vi "WebServiceFGV.vi"(7 "CMD":T5, 8 "error in (no error)":errorcluster, 9 "ClientTimeout(s)(30)":dbl=30.0 format="%#_13g", 10 "ClientName":string, 11 "SRListIn":T3=[{"SR#"=0.0, "Group"="", "Owner"="", "Problem Summary"="", "Last Updated"=timestamp(0 s since 1904-01-01), "Customer First Name"="", "Customer Last Name"="", "Company"="", "Created On"=timestamp(0 s since 1904-01-01), "SR Type"="", "Status"="", "Service Level"="", "Channel"="", "Days Open"=0.0}] {"SR#" format="%#_10g"}) -> (0 "error out":errorcluster, 2 "ClientList":T1, 3 "SRListOut":T3 {"SR#" format="%#_10g"})   [LabVIEW 2017, in "Server.lvlib" / "WebServiceCommunication.lvlib"]
uses:
  WebServiceCommunication.lvlib
  WebServiceFGVcommands.ctl
  TypeDefs/SR List.ctl
  TypeDefs/SR Data.ctl
  TypeDefs/ClientList.ctl
  TypeDefs/ClientData.ctl
  WebServiceData.ctl
  Server.lvlib
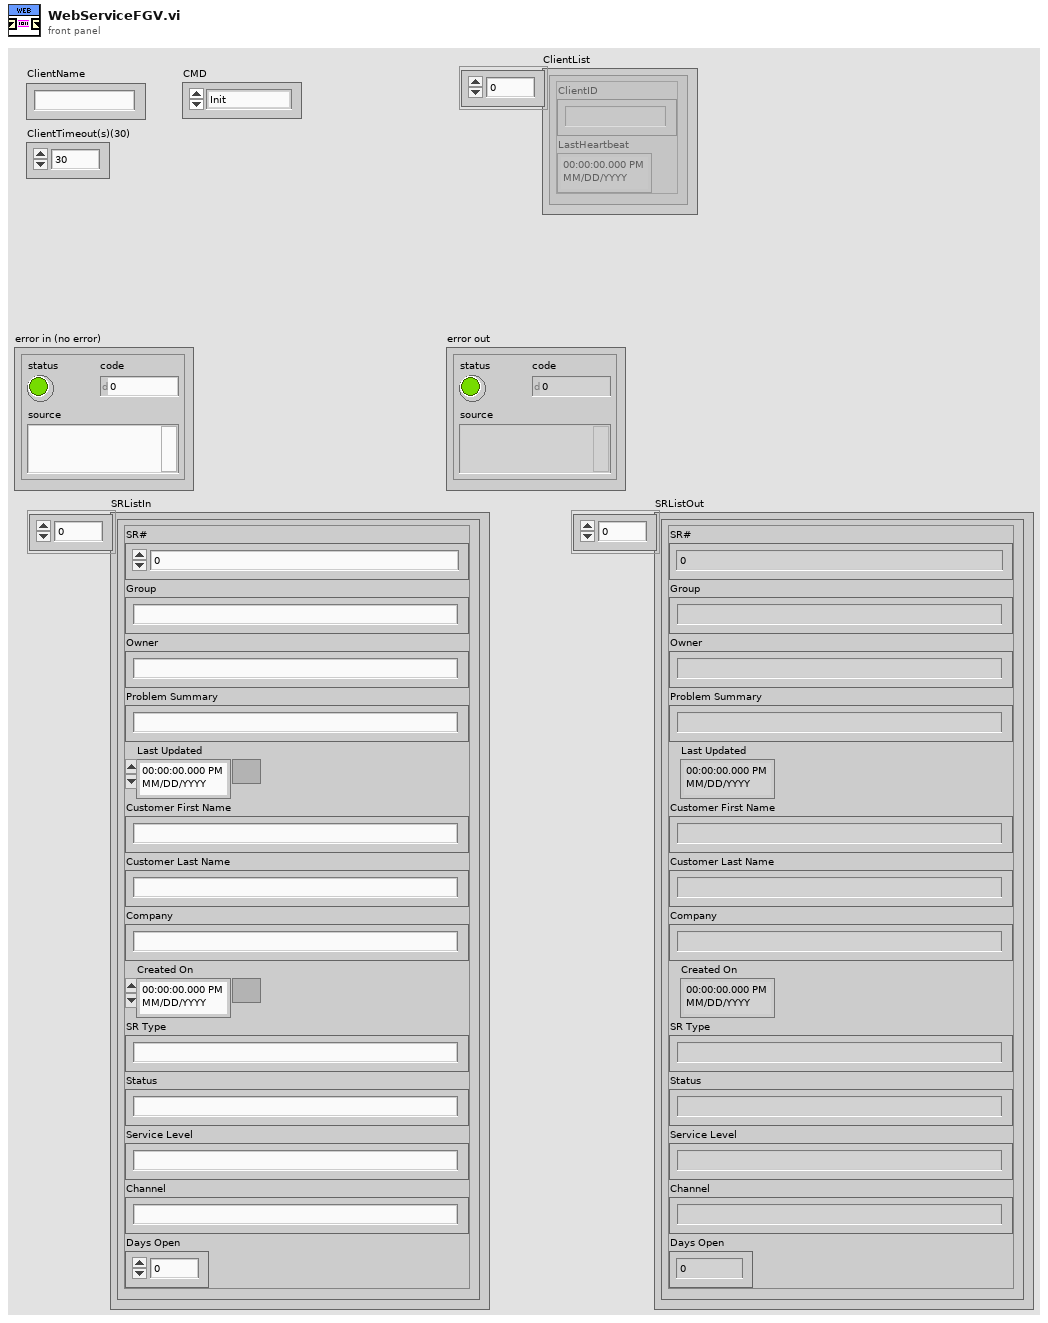
[diagram p1: front panel]
types:
  T1 = typedef "Server.lvlib/ClientList.ctl" = T2[]
  T2 = typedef "Server.lvlib/ClientData.ctl" = cluster{"ClientID":string, "LastHeartbeat":timestamp}
  T3 = typedef "Server.lvlib/SR List.ctl" = T4[]
  T4 = typedef "Server.lvlib/SR Data.ctl" = cluster{"SR#":dbl, "Group":string, "Owner":string, "Problem Summary":string, "Last Updated":timestamp, "Customer First Name":string, "Customer Last Name":string, "Company":string, "Created On":timestamp, "SR Type":string, "Status":string, "Service Level":string, "Channel":string, "Days Open":dbl}
  T5 = typedef "Server.lvlib/WebServiceCommunication.lvlib/WebServiceFGVcommands.ctl" = enum16{"Init", "Reset", "Heartbeat", "GetSRs", "SetSRs", "CheckClients", "GetClients"}
  T6 = typedef "Server.lvlib/WebServiceCommunication.lvlib/WebServiceData.ctl" = cluster{"SRList":T3, "ClientList":T1}
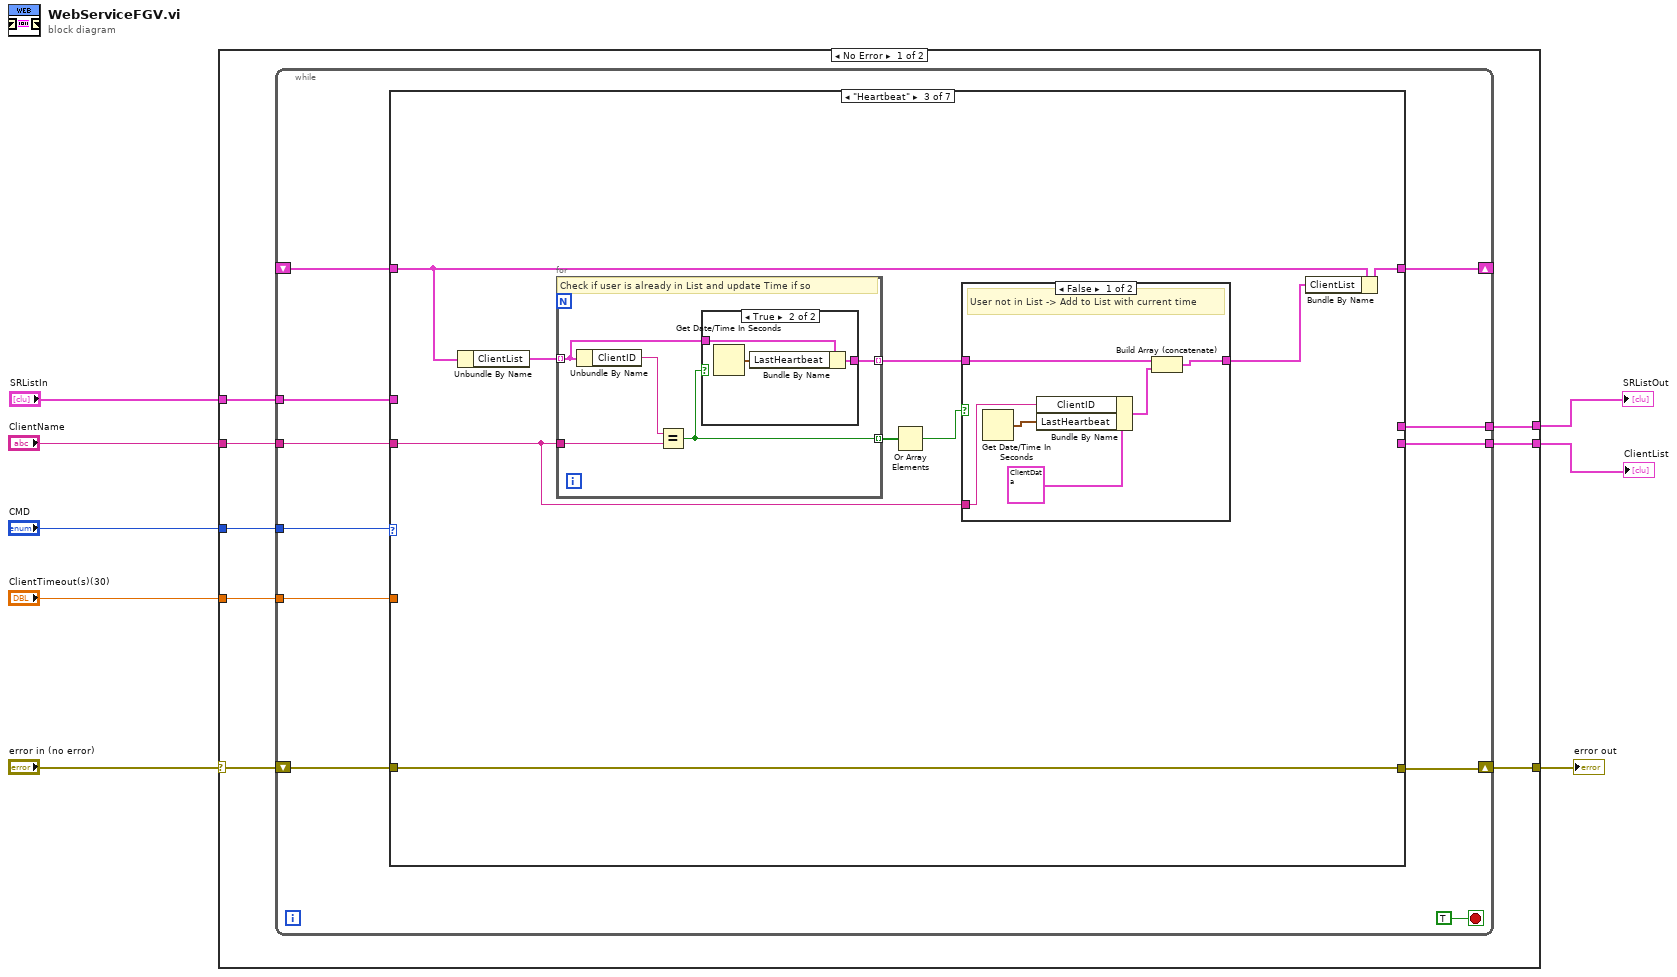
[diagram p0: block diagram]
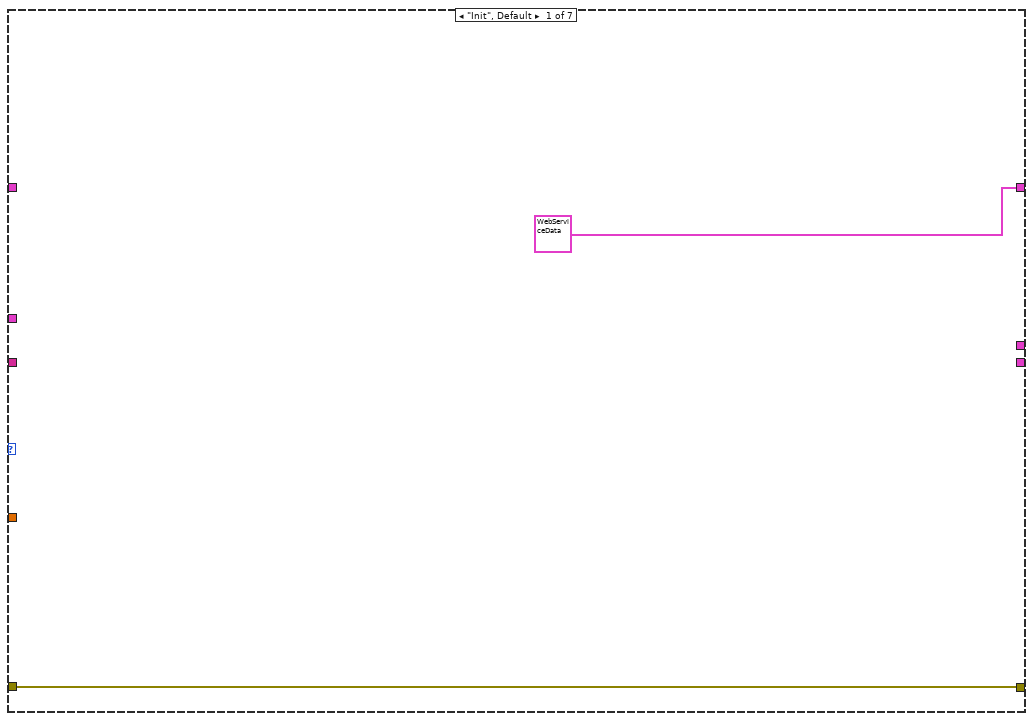
[diagram p2: hidden frame]
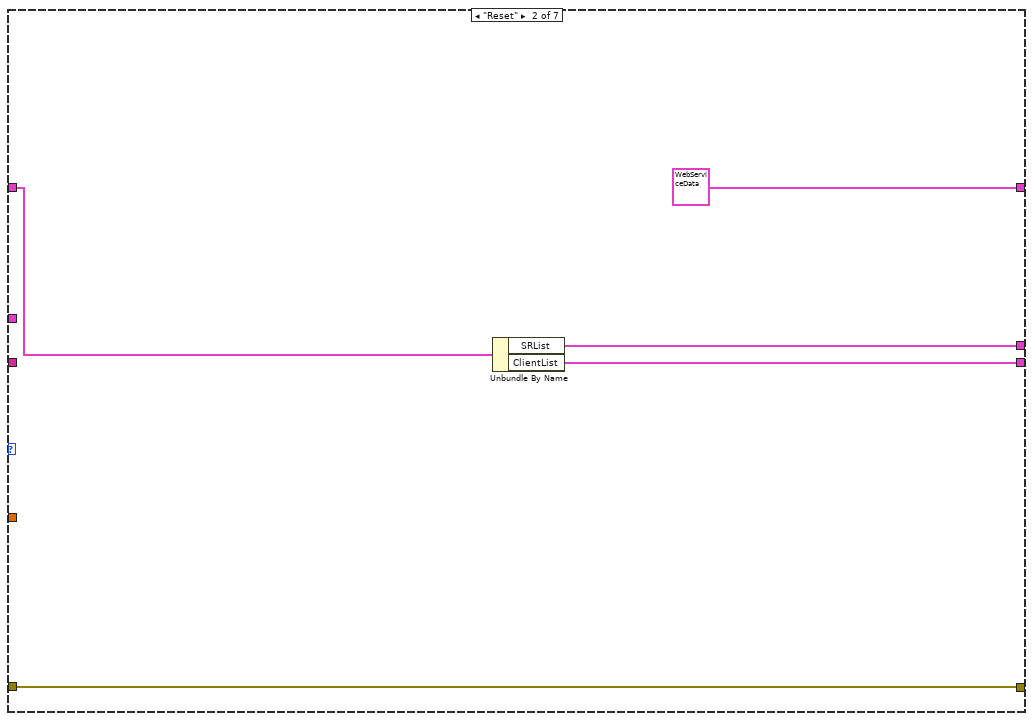
[diagram p3: hidden frame]
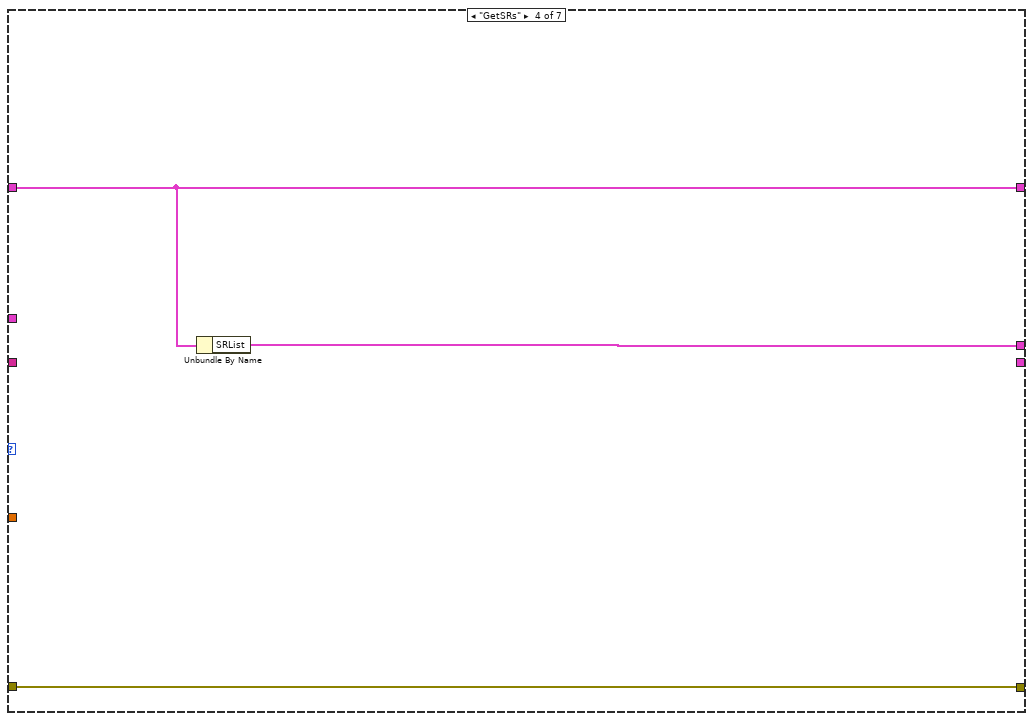
[diagram p6: hidden frame]
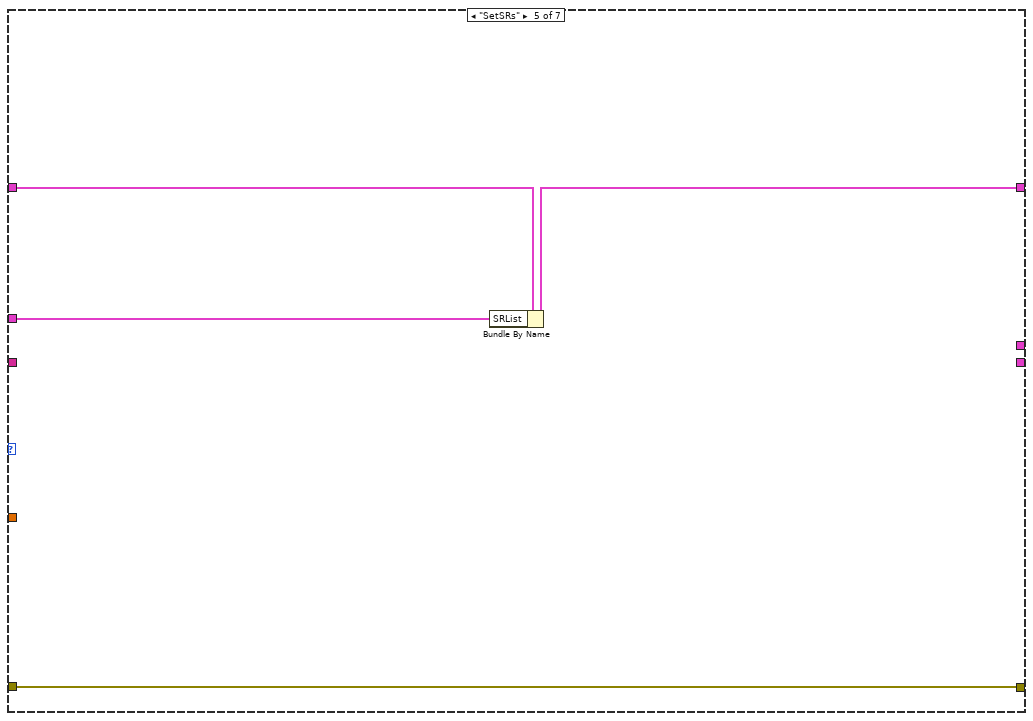
[diagram p7: hidden frame]
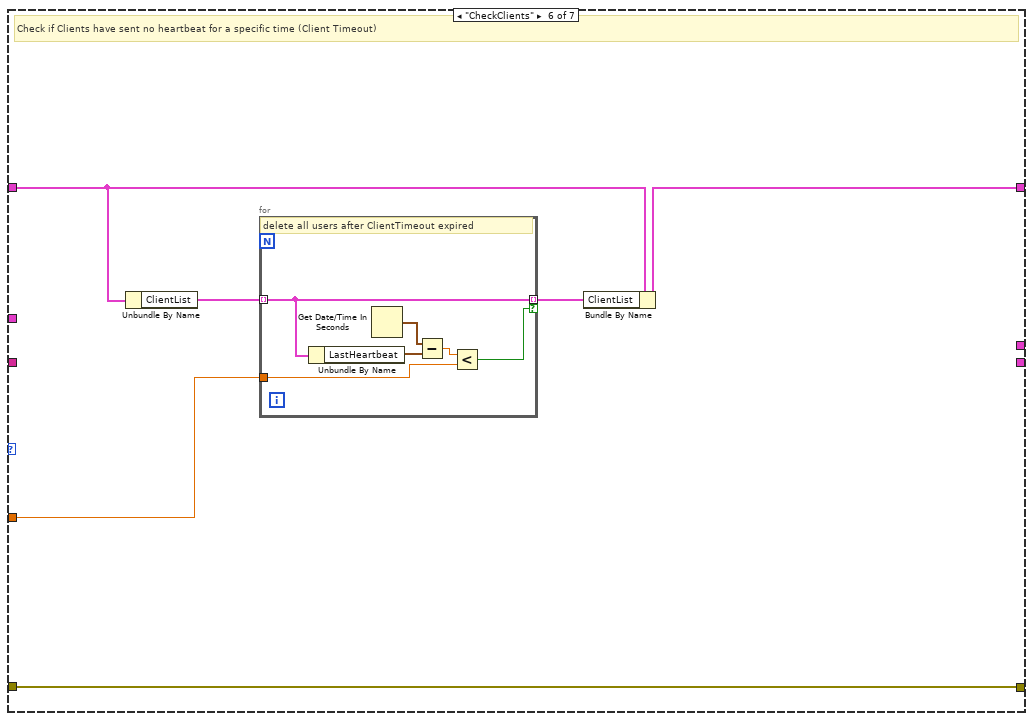
[diagram p8: hidden frame]
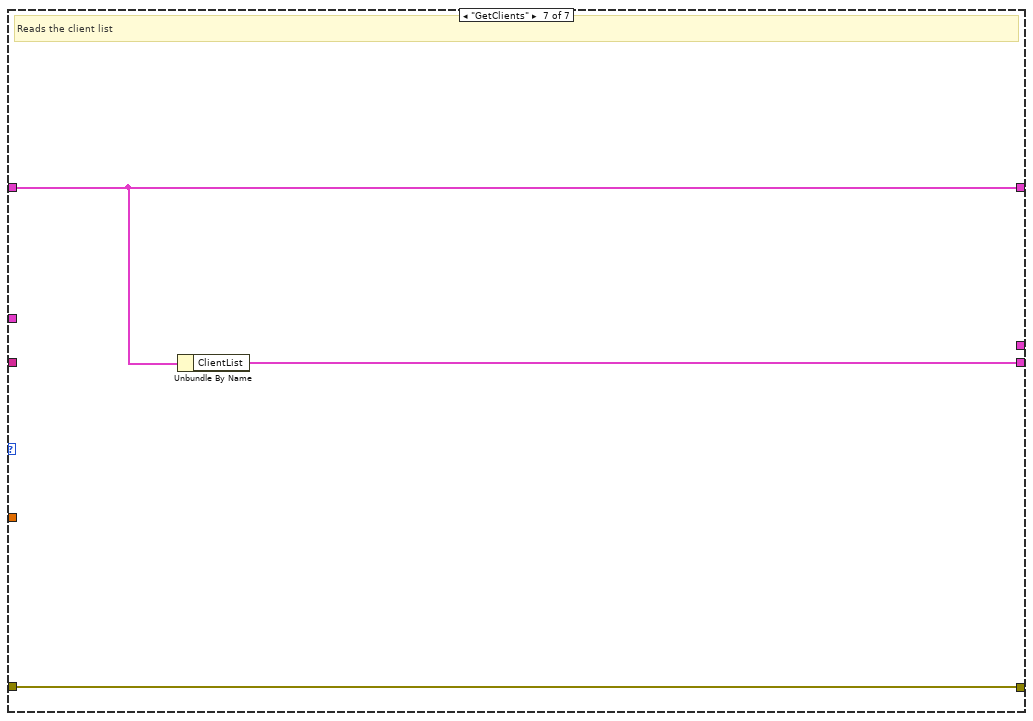
[diagram p9: hidden frame]
diagram:
  n1 = case shown="No Error" "error in (no error)" {
    selector: "error in (no error)" -> [w14 w82]
    tunnel: "CMD" -> [w16 _]
    tunnel: [w15 w82] -> w7
    tunnel: [w13 _] -> w2
    tunnel: [w12 _] -> w1
    tunnel: "SRListIn" -> [w11 _]
    tunnel: "ClientName" -> [w10 _]
    tunnel: "ClientTimeout(s)(30)" -> [w9 _]
    frame No Error {
      n2 = while {
        shift-right: [w25] -> _
        shift-left: _ -> [w24]
        tunnel: w16 -> [w26]
        shift-right: [w22] -> w15
        shift-left: w14 -> [w23]
        tunnel: [w21] -> w13
        tunnel: [w20] -> w12
        tunnel: w11 -> [w19]
        tunnel: w10 -> [w18]
        tunnel: w9 -> [w17]
        stop <- TRUE stop-if-true
        n3 = case shown="\"Heartbeat\"" w26 {
          tunnel: [T6 {"SRList"=[{"SR#"=0.0, "Group"="", "Owner"="", "Problem Summary"="", "Last Updated"=timestamp(0 s since 1904-01-01), "Customer First Name"="", "Customer Last Name"="", "Company"="", "Created On"=timestamp(0 s since 1904-01-01), "SR Type"="", "Status"="", "Service Level"="", "Channel"="", "Days Open"=0.0}], "ClientList"=[]} ("WebServiceData") T6 {"SRList"=[{"SR#"=0.0, "Group"="", "Owner"="", "Problem Summary"="", "Last Updated"=timestamp(0 s since 1904-01-01), "Customer First Name"="", "Customer Last Name"="", "Company"="", "Created On"=timestamp(0 s since 1904-01-01), "SR Type"="", "Status"="", "Service Level"="", "Channel"="", "Days Open"=0.0}], "ClientList"=[]} ("WebServiceData") w36 w61 w64 w70 w80] -> w25
          tunnel: w24 -> [_ w32 w42 w61 w66 w71 w80]
          tunnel: [w28 w34 w43 w62 w65 w72 w81] -> w22
          tunnel: w23 -> [w28 w34 w43 w62 w65 w72 w81]
          tunnel: [_ w31 _ w60 _ _ _] -> w21
          tunnel: [_ w30 _ _ _ _ w79] -> w20
          tunnel: w19 -> [_ _ _ _ w63 _ _]
          tunnel: w18 -> [_ _ w38 _ _ _ _]
          tunnel: w17 -> [_ _ _ _ _ w68 _]
          frame "Init", Default {
          }
          frame "Reset" {
            n4 = Unbundle By Name(w32) -> ("SRList"=w31:T3, "ClientList"=w30:T1)
          }
          frame "Heartbeat" {
            n5 = Unbundle By Name(w42) -> ("ClientList"=w41:T1)
            n6 = for {
              tunnel: w41 -> [w53] mode=indexing
              tunnel: w38 -> [w55]
              tunnel: [w52] -> w40 mode=indexing
              tunnel: [w51] -> w39 mode=indexing
              # "Check if user is already in List and update Time if so"
              n7 = Unbundle By Name(w53) -> ("ClientID"=w54:string)
              n8 = Equal?(x=w54, y=w55) -> (x = y?=w52:bool)
              n9 = case shown="True" w52 {
                tunnel: w53 -> [w56 w59]
                tunnel: [w56 w58] -> w51
                frame False {
                }
                frame True {
                  n10 = Get Date/Time In Seconds() -> (seconds since 1Jan1904=w57:timestamp)
                  n11 = Bundle By Name(cluster=w59, "LastHeartbeat"=w57) -> (w58:T2)
                }
              }
            }
            n12 = Or Array Elements(Boolean array=w40) -> (logical OR=w37:bool)
            n13 = case shown="False" w37 {
              tunnel: w39 -> [w49 w50]
              tunnel: w38 -> [w47 _]
              tunnel: [w46 w50] -> w35
              frame False {
                # "User not in List -> Add to List with current time"
                n14 = Get Date/Time In Seconds() -> (seconds since 1Jan1904=w45:timestamp)
                n15 = Bundle By Name(cluster=T2 {"ClientID"="", "LastHeartbeat"=timestamp(0 s since 1904-01-01)} ("ClientData"), "ClientID"=w47, "LastHeartbeat"=w45) -> (w48:T2)
                n16 = Build Array (concatenate)(w49, w48) -> (w46:T2[])
              }
              frame True {
              }
            }
            n17 = Bundle By Name(cluster=w42, "ClientList"=w35) -> (w36:T6)
          }
          frame "GetSRs" {
            n18 = Unbundle By Name(w61) -> ("SRList"=w60:T3)
          }
          frame "SetSRs" {
            n19 = Bundle By Name(cluster=w66, "SRList"=w63) -> (w64:T6)
          }
          frame "CheckClients" {
            # "Check if Clients have sent no heartbeat for a specific time (Client Timeout)"
            n20 = Unbundle By Name(w71) -> ("ClientList"=w69:T1)
            n21 = for {
              tunnel: w69 -> [w74] mode=indexing
              tunnel: w68 -> [w75]
              tunnel: [w74] -> w67 mode=indexing if=w73
              # "delete all users after ClientTimeout expired"
              n22 = Unbundle By Name(w74) -> ("LastHeartbeat"=w77:timestamp)
              n23 = Get Date/Time In Seconds() -> (seconds since 1Jan1904=w78:timestamp)
              n24 = Subtract(x=w78, y=w77) -> (x-y=w76:dbl)
              n25 = Less?(x=w76, y=w75) -> (x < y?=w73:bool)
            }
            n26 = Bundle By Name(cluster=w71, "ClientList"=w67) -> (w70:T6)
          }
          frame "GetClients" {
            # "Reads the client list"
            n27 = Unbundle By Name(w80) -> ("ClientList"=w79:T1)
          }
        }
      }
    }
    frame Error {
    }
  }
  "error out" <- w7
  "SRListOut" <- w2
  "ClientList" <- w1
